vi "Read Array of Data Files.vi"(0 "Data Files":path[](array[path])) -> (1 "Merged Channels":string[](array[string]), 2 "Data Array":string[][](array[string]))   [LabVIEW 2022 SP3]
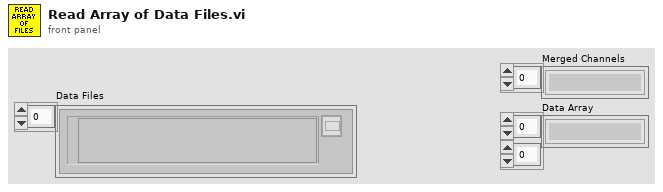
[diagram p1: front panel]
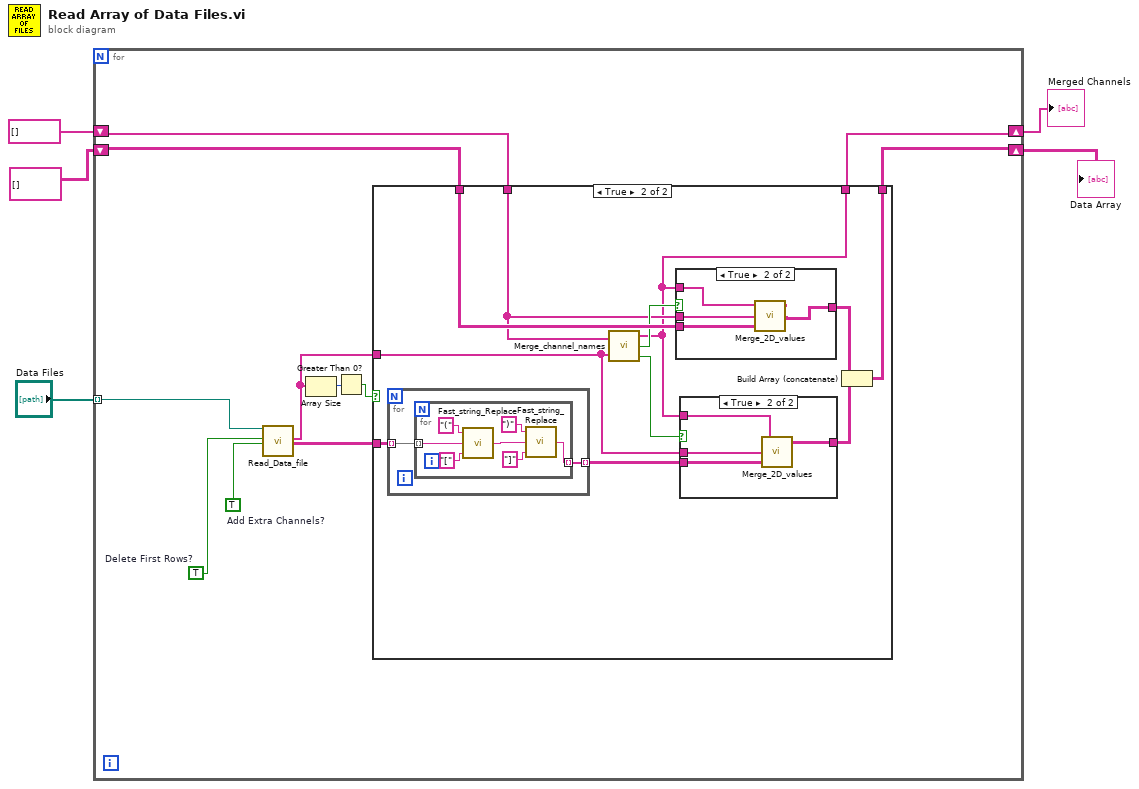
[diagram p0: block diagram]
diagram:
  n1 = for {
    shift-right: [w15] -> w2
    shift-left: string[] [] ("Merged Channels") -> [w14]
    shift-right: [w16] -> w1
    shift-left: string[][] [] -> [w13]
    tunnel: "Data Files" -> [w6] mode=indexing
    w7 = TRUE  # Delete First Rows?
    w10 = TRUE  # Add Extra Channels?
    n2 = call "Read_Data_file.vi"("Results file"=w6, "Delete First Rows?"=w7, "Add Extra Channels?"=w10) -> ("Ch names Out"=w11:string[], "Channel Values Out"=w9:string[][])  [unwired: 4 in, 11 out]
    n3 = Array Size(array=w11) -> (size(s)=w12:i32)
    n4 = Greater Than 0?(x=w12) -> (x > 0?=w8:bool)
    n5 = case shown="True" w8 {
      tunnel: w13 -> [w17 w29]
      tunnel: w14 -> [w18 w24]
      tunnel: w9 -> [_ w22]
      tunnel: [w17 w20] -> w16
      tunnel: [w18 w19] -> w15
      tunnel: w11 -> [_ w23]
      frame False {
      }
      frame True {
        n6 = for {
          tunnel: w22 -> [w31] mode=indexing
          tunnel: [w30] -> w21 mode=indexing
          n7 = for {
            tunnel: w31 -> [w33] mode=indexing
            tunnel: [w32] -> w30 mode=indexing
            n8 = call "Fast_string_Replace.vi"("Replace match with:"="[", "Input String"=w33, "matchThis"="(" ("regular expression")) -> ("Output String"=w34:string)  [unwired: 1 in, 1 out]
            n9 = call "Fast_string_Replace.vi"("Replace match with:"="]", "Input String"=w34, "matchThis"=")" ("regular expression")) -> ("Output String"=w32:string)  [unwired: 1 in, 1 out]
          }
        }
        n10 = call "Merge_channel_names.vi"("Preferred Channel array"=w24, "Channel array"=w23) -> ("Merged Channels"=w19:string[], "Preferred Channels Changed?"=w26:bool, "Channel Array Changed?"=w27:bool)
        n11 = case shown="True" w26 {
          tunnel: w29 -> [w44 w46]
          tunnel: w24 -> [_ w48]
          tunnel: [w44 w45] -> w25
          tunnel: w19 -> [_ w47]
          frame False {
          }
          frame True {
            n12 = call "Merge_2D_values.vi"("Values In"=w46, "Present Channels"=w48, "Desired Channels"=w47) -> ("Values Out"=w45:string[][])
          }
        }
        n13 = case shown="True" w27 {
          tunnel: [w39 w43] -> w28
          tunnel: w23 -> [_ w42]
          tunnel: w21 -> [w39 w41]
          tunnel: w19 -> [_ w40]
          frame False {
          }
          frame True {
            n14 = call "Merge_2D_values.vi"("Values In"=w41, "Present Channels"=w42, "Desired Channels"=w40) -> ("Values Out"=w43:string[][])
          }
        }
        n15 = Build Array (concatenate)(w25, w28) -> (w20:string[][])
      }
    }
  }
  "Merged Channels" <- w2
  "Data Array" <- w1
